vi "LWXPS_ISRCorrectorCompensateOverrunNumberGet.vi"(8 "LabVIEW error IN":errorcluster, 11 "XPS Reference IN":refnum<k24>) -> (0 "Corrector Overrun Compensation Miss Number":i32, 1 "Corrector Overrun Compensation Number":i32, 2 "XPS Error String":string, 3 "Returned error code":i32, 4 "LabVIEW error OUT":errorcluster, 5 "XPS Reference OUT":refnum<k24>)   [LabVIEW 2014]
uses:
  D:/XPSQ8_LabView_Library/Development/Source/Dll/Newport.XPS.CommandInterface.dll
  Dll/Newport.XPS.CommandInterface.dll
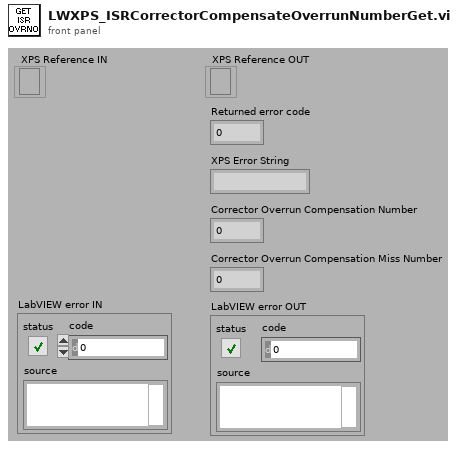
[diagram p1: front panel]
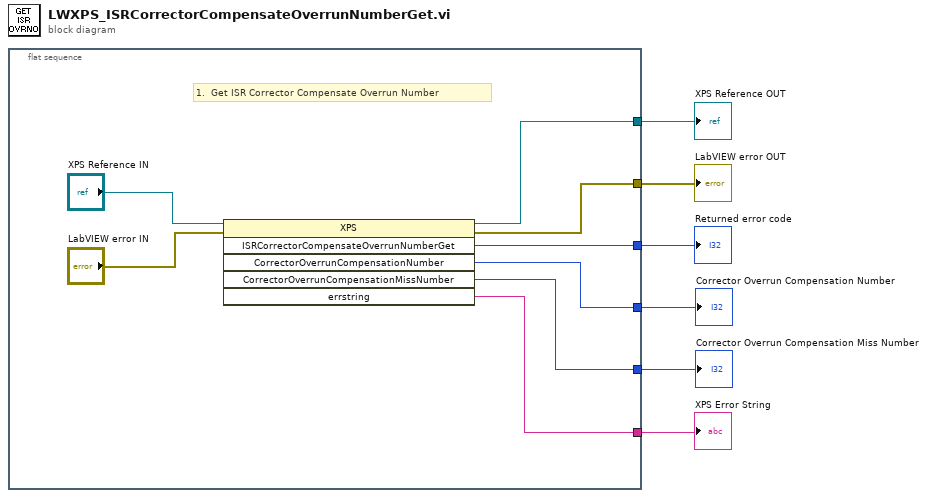
[diagram p0: block diagram]
diagram:
  n1 = flat-sequence {
    tunnel: [w12] -> w6
    tunnel: [w14] -> w5
    tunnel: [w11] -> w4
    tunnel: [w10] -> w2
    tunnel: [w8] -> w1
    tunnel: [w7] -> w3
    frame #0 {
      # "1.  Get ISR Corrector Compensate Overrun Number"
      n2 = invoke class="XPS" method="ISRCorrectorCompensateOverrunNumberGet"(reference="XPS Reference IN", error in="LabVIEW error IN") -> (reference out=w12:refnum<k24>, error out=w14:errorcluster, "ISRCorrectorCompensateOverrunNumberGet"=w11:i32, "CorrectorOverrunCompensationNumber"=w10:i32, "CorrectorOverrunCompensationMissNumber"=w8:i32, "errstring"=w7:string)  [unwired: 4 in]
    }
  }
  "XPS Reference OUT" <- w6
  "LabVIEW error OUT" <- w5
  "Returned error code" <- w4
  "XPS Error String" <- w3
  "Corrector Overrun Compensation Number" <- w2
  "Corrector Overrun Compensation Miss Number" <- w1
